vi "Get Lockin Channels.vi"(8 "error in (no error)":errorcluster, 11 "MeasurementSMO in":refnum<class "MeasurementSMO.lvclass">) -> (0 "error out":errorcluster, 1 "Channels":i32[](array[numeric]), 2 "size(s)":i32, 3 "MeasurementSMO out":refnum<class "MeasurementSMO.lvclass">)   [LabVIEW 2019, in "MeasurementSMO.lvclass"]
uses:
  MeasurementSMO.lvclass
  MeasurementSMO.lvclass/MeasurementSMO.ctl
  <userlib>/LevyLab/Lockin-Multichannel/Instrument.Lockin/Instrument.Lockin.lvclass
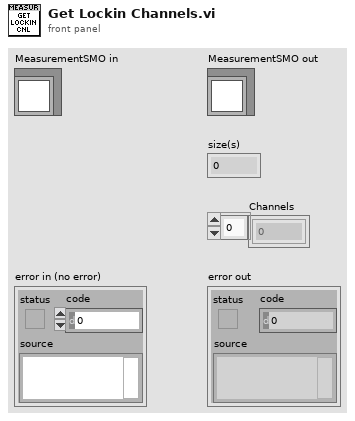
[diagram p1: front panel]
types:
  T1 = typedef "Instrument.DAQ.lvclass/AO.Channel--Cluster--Array.ctl" = T2[]
  T2 = typedef "Instrument.DAQ.lvclass/AO.Channel--Cluster.ctl" = cluster{"Enable?":bool, "Channel":i32, "Amplitude":dbl, "Offset":dbl, "Frequency":dbl, "Phase":dbl, "Function":T3, "Sweeping?":bool}
  T3 = typedef "Instrument.DAQ.lvclass/AO.Channel.Function--Enum.ctl" = enum16{"Sine", "Triangle", "Square"}
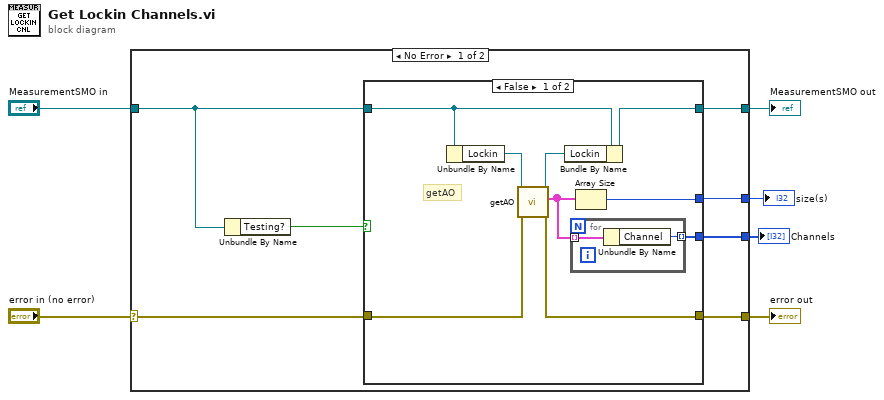
[diagram p0: block diagram]
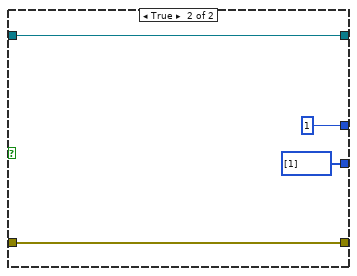
[diagram p2: hidden frame]
diagram:
  n1 = case shown="No Error" "error in (no error)" {
    selector: "error in (no error)" -> [w12 w30]
    tunnel: [w11 w30] -> w5
    tunnel: [w13 w29] -> w3
    tunnel: "MeasurementSMO in" -> [w9 w29]
    tunnel: [w10 _] -> w2
    tunnel: [w7 _] -> w1
    frame No Error {
      n2 = Unbundle By Name(w9) -> ("Testing?"=w8:bool)
      n3 = case shown="False" w8 {
        tunnel: [w22 w28] -> w13
        tunnel: w9 -> [w21 w28]
        tunnel: w12 -> [w14 w26]
        tunnel: [w15 w26] -> w11
        tunnel: [w20 1] -> w10
        tunnel: [w19 i32[] [1]] -> w7
        frame False {
          # "getAO"
          n4 = Unbundle By Name(w21) -> ("Lockin"=w18:refnum<class "Instrument.Lockin.lvclass">)
          n5 = call <userlib>:"getAO.vi"("error in (no error)"=w14, "Instrument.Lockin in"=w18) -> ("error out"=w15:errorcluster, "AOconfig"=w16:T1, "Instrument.Lockin out"=w17:refnum<class "Instrument.Lockin.lvclass">)  [unwired: 7 in]
          n6 = Bundle By Name(cluster=w21, "Lockin"=w17) -> (w22:refnum<class "MeasurementSMO.lvclass">)
          n7 = for {
            tunnel: w16 -> [w24] mode=indexing
            tunnel: [w23] -> w19 mode=indexing
            n8 = Unbundle By Name(w24) -> ("Channel"=w23:i32)
          }
          n9 = Array Size(array=w16) -> (size(s)=w20:i32)
        }
        frame True {
        }
      }
    }
    frame Error {
    }
  }
  "error out" <- w5
  "MeasurementSMO out" <- w3
  "size(s)" <- w2
  "Channels" <- w1
